vi "PID.vi"(0 "Z":dbl, 1 "Xclosest":dbl, 2 "ErrorIn":dbl[](array[numeric]), 3 "Yclosest":dbl, 4 "Zclosest":dbl, 5 "Kp":dbl, 6 "Ki":dbl, 7 "IntegralIn":dbl[](array[numeric]), 8 "Y":dbl, 9 "Kd":dbl, 12 "X":dbl, 13 "deltaT":dbl) -> (20 "FPID":dbl[](array[numeric]), 21 "IntegralOut":dbl[](array[numeric]), 25 "ErrorOut":dbl[](array[numeric]))   [LabVIEW 2020]
uses:
  <vilib>/imath/engines/lvmath2/RunTimeEngine/ArithmeticOperatorToken/NIMS_ArithmeticOperator_plus.vi
  <instcachedir>/0/NIMS_ArithmeticOperator_plus_54468E2FAC2848C4BF0D457641184E60.lvgen/NIMS_ArithmeticOperator_plus_54468E2FAC2848C4BF0D457641184E60_004.vi
  <vilib>/imathl/engines/lvmath/Functions/Error Handling/Create Error.vi
  <vilib>/imath/engines/lvmath2/RunTimeEngine/ArithmeticOperatorToken/NIMS_ArithmeticOperator_minus.vi
  <instcachedir>/0/NIMS_ArithmeticOperator_minus_822089A08BE049DB927E6BEA78E100F1.lvgen/NIMS_ArithmeticOperator_minus_822089A08BE049DB927E6BEA78E100F1_003.vi
  <vilib>/imath/engines/lvmath2/RunTimeEngine/ErrorHandling/NIMS_Create Error From Enums.vi
  <vilib>/imath/engines/lvmath2/RunTimeEngine/NodeEndStatement/NIMS_NodeEndStatement_Output.vi
  <instcachedir>/0/NIMS_NodeEndStatement_Output_53EC0D466D134D7ABD903AC30B43404B.lvgen/NIMS_NodeEndStatement_Output_53EC0D466D134D7ABD903AC30B43404B_005.vi
  <vilib>/imath/engines/lvmath2/RunTimeEngine/ErrorHandling/NIMS_Finalize Error.vi
panel:
  # "Inputs"
  # "Outputs"
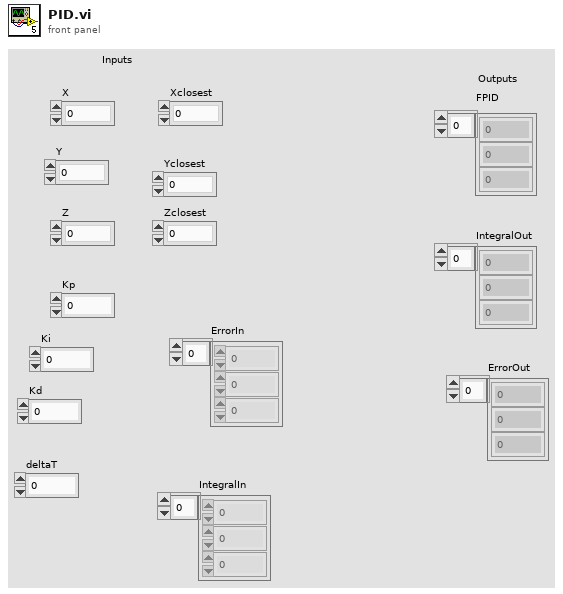
[diagram p1: front panel]
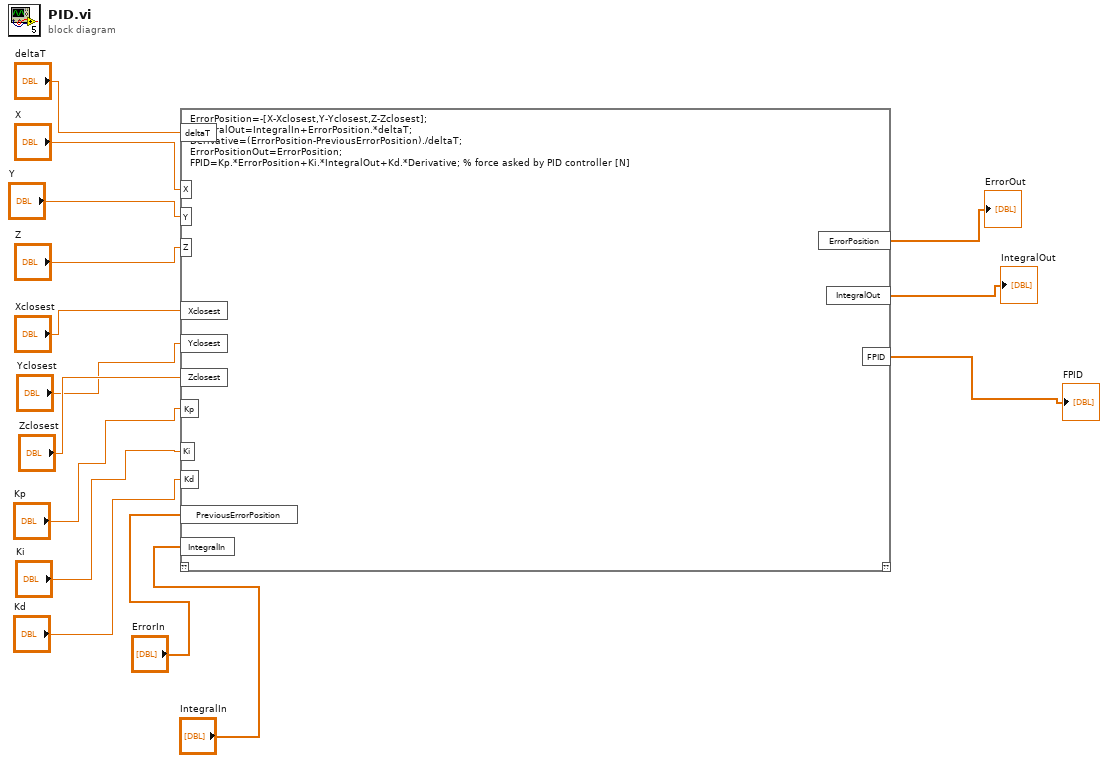
[diagram p0: block diagram]
diagram:
  n1 = mathscript code="ErrorPosition=-[X-Xclosest,Y-Yclosest,Z-Zclosest];\nIntegralOut=IntegralIn+ErrorPosition.*deltaT;\nDerivative=(ErrorPosition-PreviousErrorPosition)./deltaT;\nErrorPositionOut=ErrorPosition;\nFPID=Kp.*ErrorPosition+Ki.*IntegralOut+Kd.*Derivative; % force asked by PID controller [N]"("X"="X", "Y"="Y", "Z"="Z", "Xclosest"="Xclosest", "Yclosest"="Yclosest", "Zclosest"="Zclosest", "Kp"="Kp", "Ki"="Ki", "Kd"="Kd", "deltaT"="deltaT", "PreviousErrorPosition"="ErrorIn", "IntegralIn"="IntegralIn") -> ("ErrorPosition"=→"ErrorOut":dbl[], "IntegralOut"=→"IntegralOut":dbl[], "FPID"=→"FPID":dbl[])  [unwired: 1 in, 1 out]
